vi "Go Back.vi"(8 "Error In":errorcluster, 11 "object in":refnum<class "WebView.lvclass">) -> (0 "Error Out":errorcluster, 3 "object out":refnum<class "WebView.lvclass">)   [LabVIEW 2024, in "WebView.lvclass"]
uses:
  WebView.lvclass
  <vilib>/sklein/WebView2/Libs/Microsoft.Web.WebView2.Core.dll
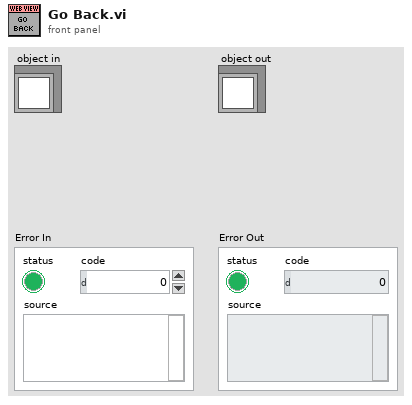
[diagram p1: front panel]
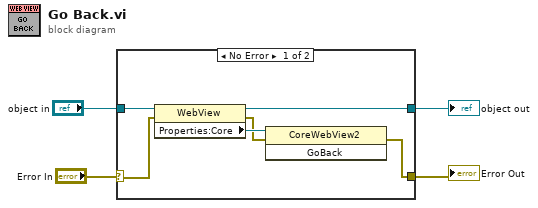
[diagram p0: block diagram]
diagram:
  n1 = case shown="No Error" "Error In" {
    selector: "Error In" -> [w8 w12]
    tunnel: [w5 w12] -> w3
    tunnel: [w9 w11] -> w1
    tunnel: "object in" -> [w10 w11]
    frame No Error {
      n2 = property class="WebView"(reference=w10, error in=w8) -> (reference out=w9:refnum<class "WebView.lvclass">, error out=w6:errorcluster, "Properties:Core"=w7:refnum<k24>)
      n3 = invoke class="CoreWebView2" method="GoBack"(reference=w7, error in=w6) -> (error out=w5:errorcluster)  [unwired: 1 in, 2 out]
    }
    frame Error {
    }
  }
  "Error Out" <- w3
  "object out" <- w1
